vi "RT Loop - Data Acquisition - NLHQ.vi"(8 "error in (no error)":errorcluster caption="错误输入（无错误）", 11 "Message Queues":T1 caption="消息队列") -> (0 "error out":errorcluster caption="错误输出")   [LabVIEW 2015]
uses:
  Support VIs/Message Queue/All Real-Time Message Queues.ctl
  Support VIs/Message Queue/Message Cluster.ctl
  Globals/Global - Monitoring Variables.vi
  Globals/Global - Configuration Options.vi
  Support VIs/Message Queue/Message Queue.lvlib
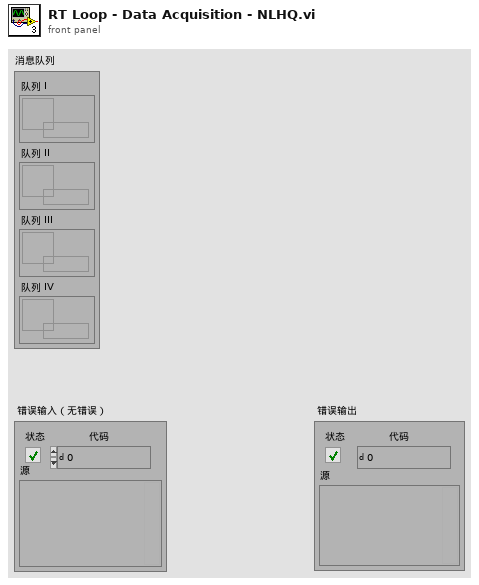
[diagram p1: front panel]
types:
  T1 = typedef "Message Queue.lvlib/All Real-Time Message Queues.ctl" = cluster{"Queue I":refnum<queue>, "Queue II":refnum<queue>, "Queue III":refnum<queue>, "Queue IV":refnum<queue>}
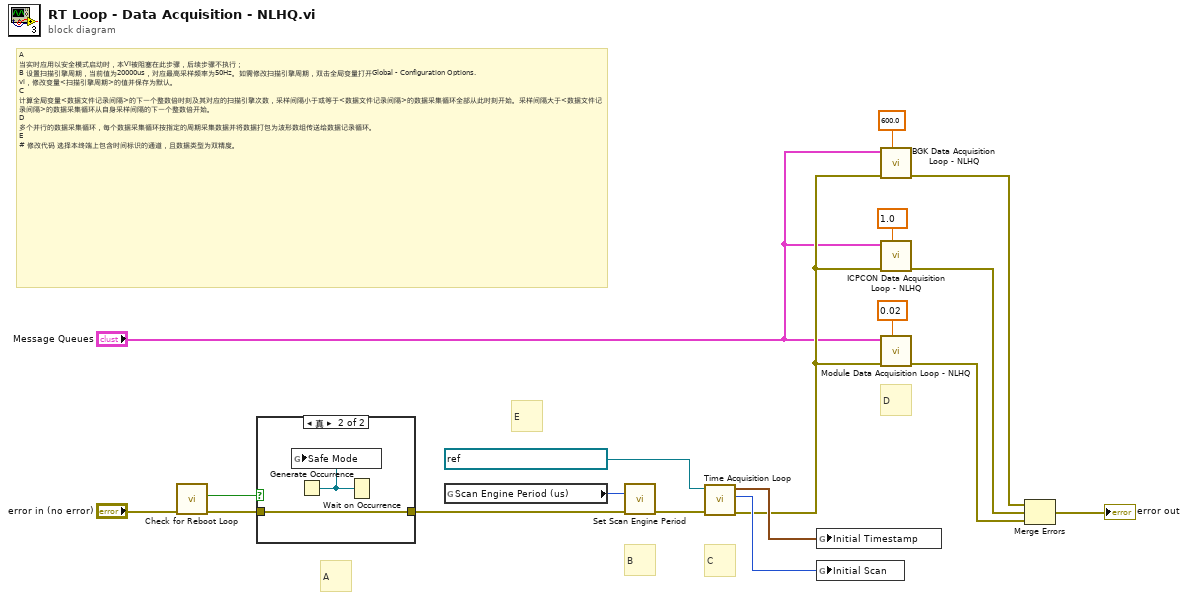
[diagram p0: block diagram]
diagram:
  # "E"
  # "A\n当实时应用以安全模式启动时，本VI被阻塞在此步骤，后续步骤不执行；\nB 设置扫描引擎周期，当前值为20000us，对应最高采样频率为50Hz。如需修改扫描引擎周期，双击全局变量打开Global - Configuration Options.vi，修改变量<扫描引擎周期>的值并保存为默认。\nC\n计算全局变量<数据文件记录间隔>的下一个整数倍时刻及其对应的扫描引擎次数，采样间隔小于或等于<数据文件记录间隔>的数据采集循环全部从此时刻开始。采样间隔大于<数据文件记录间隔>的数据采集循环从自身采样间隔的下一个整数倍开始。\nD\n多个并行的数据采集循环，每个数据采集循环按指定的周期采集数据并将数据打包为波形数组传送给数据记录循环。\nE\n# 修改代码 选择本终端上包含时间标识的通道，且数据类型为双精度。"
  # "D"
  # "C"
  # "B"
  # "A"
  n1 = call "Check for Reboot Loop.vi"("error in (no error)"="error in (no error)") -> ("error out"=w15:errorcluster, "Start in Safe Mode?"=w16:bool)  [unwired: 9 in]
  n2 = case shown="真" w16 {
    tunnel: w15 -> [w19 w21]
    tunnel: [w19 w21] -> w12
    frame False {
    }
    frame True {
      n3 = Generate Occurrence() -> (w20:refnum<k4>)
      n4 = global write "Global - Monitoring Variables.vi" "Safe Mode"(w20) -> ()
      n5 = Wait on Occurrence(2:w20) -> ()  [unwired: 2 in, 1 out]
    }
  }
  n6 = global read "Global - Configuration Options.vi" "Scan Engine Period (us)"() -> (w10:u32)
  n7 = call <vilib>:"Set Scan Engine Period.vi"("scan period (uSec)"=w10, "error in (no error)"=w12) -> ("error out"=w11:errorcluster)  [unwired: 13 in]
  n8 = call "Time Acquisition Loop.vi"("shared variable ref"=refnum<k21> "ni.var.io://ni-crio-9036-nlhq/Mod1/NLHQ-X-02-A01", "error in (no error)"=w11) -> ("Timestamp"=w14:timestamp, "Scan Engine Time"=w13:i64, "error out"=w5:errorcluster)  [unwired: 6 in]
  n9 = global write "Global - Monitoring Variables.vi" "Initial Timestamp"(w14) -> ()
  n10 = global write "Global - Monitoring Variables.vi" "Initial Scan"(w13) -> ()
  n11 = call "BGK Data Acquisition Loop - NLHQ.vi"("Period (s)"=600.0, "error in (no error)"=w5, "Message Queues"="Message Queues") -> ("error out"=w4:errorcluster)  [unwired: 8 in]
  n12 = call "ICPCON Data Acquisition Loop - NLHQ.vi"("sampling period (s)"=1.0, "error in (no error)"=w5, "Message Queues"="Message Queues") -> ("error out"=w7:errorcluster)  [unwired: 8 in]
  n13 = call "Module Data Acquisition Loop - NLHQ.vi"("Sampling Period (S)"=0.02 ("Sampling Period(S)"), "error in (no error)"=w5, "Message Queues"="Message Queues") -> ("error out"=w9:errorcluster)  [unwired: 8 in]
  n14 = Merge Errors(w4, w7, w9) -> (→"error out":errorcluster)
